vi "PopulatePrinterInitConfigDict.vi"(8 "error in (no error)":errorcluster, 11 "TopLevel in":refnum<class "TopLevel.lvclass">) -> (0 "error out":errorcluster, 3 "TopLevel out":refnum<class "TopLevel.lvclass">)   [LabVIEW 2022 SP3, in "TopLevel.lvclass"]
uses:
  TopLevel.lvclass
  Typedefs/PrinterHeads--Enum.ctl
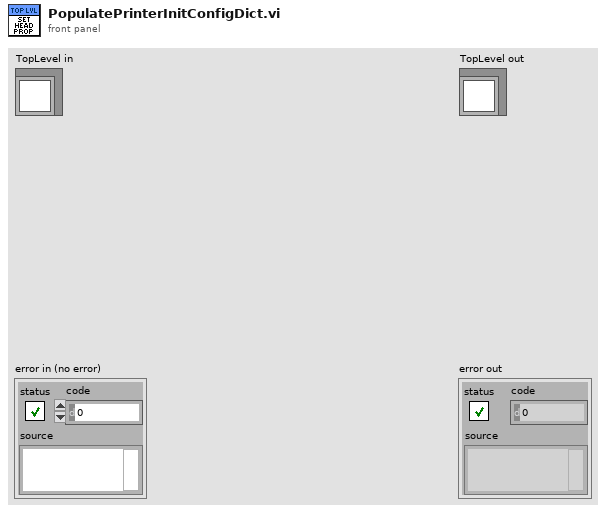
[diagram p1: front panel]
types:
  T1 = typedef "PrinterHeads--Enum.ctl" = enum16{"-1", "1", "2", "3", "4", "5", "6"}
  T2 = typedef "TD Dynamic CVT DVR--ref.ctl" = refnum<data-value>
  T3 = typedef "DLPConfig_Initialization.ctl" = cluster{"PrinterInitialization":cluster{"Printer":cluster{"#attributes":cluster{"Name":string}}, "VacPumpSet":cluster{"#attributes":cluster{"VacPumpEnable":bool, "VacPumpSpeed":dbl}}, "HIBEnable":cluster{"#attributes":cluster{"HIB1Enable":bool, "HIB2Enable":bool, "HIB3Enable":bool, "HIB4Enable":bool, "HIB5Enable":bool, "HIB6Enable":bool}}, "PrinterCompensation":T4}, "HeadSet":cluster{"HeadProperties":T5[]}, "InkSet":cluster{"Ink":T7[]}, "Troubleshooting":cluster{"PMBLogging":cluster{"#attributes":cluster{"PMBMonitorDuringPrint":bool, "PMBMonitorDuringIdle":bool, "LogSwatheInputData":bool, "LogSwatheOutputData":bool, "LogPrintheadColourPlanes":bool, "LogPMBCommunication":bool, "LogSimulatedOutput":bool, "LogAllPMBCommunicationData":bool, "LogPMBSpace":bool, "ExtendedPMBSpaceLogging":bool, "LogPMBWriteSpeed":bool, "LogUsbRetries":bool}}, "HIBLogging":cluster{"#attributes":cluster{"HIBMonitoringDuringPrint":bool, "HIBMonitoringLog":bool}}}}
  T4 = typedef "DLP2_PrinterCompensationProperties.ctl" = cluster{"#attributes":cluster{"AppName":string, "PrintWeightMultiplier":dbl, "Rotation":bool, "Driver":string, "Server":string, "Database":string, "User":string, "Password":string}}
  T5 = typedef "DLP2_PrinterHeadProperties.ctl" = cluster{"#attributes":T6}
  T6 = typedef "DLPConfig)Init_HeadPropertyAttr--Cluster.ctl" = cluster{"HeadNumber":u8, "Material":string, "HeadLocalX":dbl, "HeadLocalY":dbl, "HeadRotationAngle":dbl, "VH2L_Hi":dbl, "VH2R_Hi":dbl, "VH1LA_Hi":dbl, "VH1LB_Hi":dbl, "VH1RA_Hi":dbl, "VH1RB_Hi":dbl, "VH2L_Lo":dbl, "VH2R_Lo":dbl, "VH1LA_Lo":dbl, "VH1LB_Lo":dbl, "VH1RA_Lo":dbl, "VH1RB_Lo":dbl}
  T7 = typedef "DLP2_PrinterMaterialProperties.ctl" = cluster{"#attributes":cluster{"InkType":string, "PrePrintPurge":bool, "PurgeTime":dbl, "PurgeCount":i32, "Density":dbl, "NumberofDrops":i32, "PrintWeight":dbl, "PrintheadPrime":bool}, "Idle":cluster{"Name":string, "Heat":dbl, "Meniscus":dbl, "Recirculation":bool}[], "Process":cluster{"Name":string, "Heat":dbl, "Meniscus":dbl, "Recirculation":bool, "ColorPlane":string}[]}
  T8 = cluster{"HIB1Enable":bool, "HIB2Enable":bool, "HIB3Enable":bool, "HIB4Enable":bool, "HIB5Enable":bool, "HIB6Enable":bool}
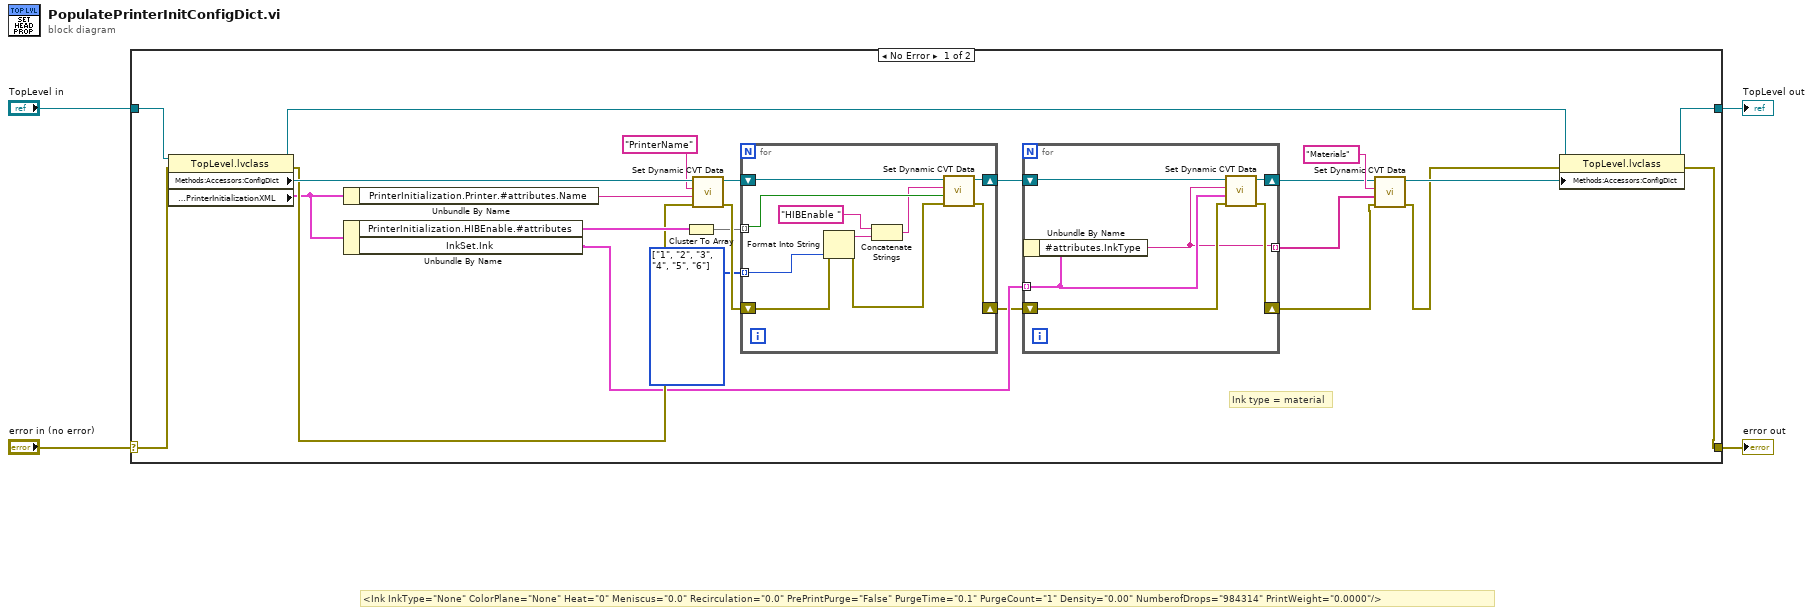
[diagram p0: block diagram]
diagram:
  # "<Ink InkType=\"None\" ColorPlane=\"None\" Heat=\"0\" Meniscus=\"0.0\" Recirculation=\"0.0\" PrePrintPurge=\"False\" PurgeTime=\"0.1\" PurgeCount=\"1\" Density=\"0.00\" NumberofDrops=\"984314\" PrintWeight=\"0.0000\"/>"
  n1 = case shown="No Error" "error in (no error)" {
    selector: "error in (no error)" -> [w23 w46]
    tunnel: [w22 w46] -> w3
    tunnel: [w27 w45] -> w1
    tunnel: "TopLevel in" -> [w24 w45]
    frame No Error {
      w14 = T1[] [enum."1", enum."2", enum."3", enum."4", enum."5", enum."6"] items=["-1", "1", "2", "3", "4", "5", "6"] ("Array")
      # "Ink type = material"
      n2 = property class="TopLevel.lvclass"(reference=w24, error in=w23) -> (reference out=w25:refnum<class "TopLevel.lvclass">, error out=w19:errorcluster, "Methods:Accessors:ConfigDict"=w28:T2, "Methods:Accessors:PrinterInitializationXML"=w16:T3)
      n3 = Unbundle By Name(w16) -> ("PrinterInitialization.Printer.#attributes.Name"=w26:string)
      n4 = Unbundle By Name(w16) -> ("PrinterInitialization.HIBEnable.#attributes"=w21:T8, "InkSet.Ink"=w12:T7[])
      n5 = Cluster To Array(cluster=w21) -> (array=w15:bool[])
      n6 = call <vilib>:"Set Dynamic CVT Data.vi"("error in (no error)"=w19, "value"=w26, "DataName"="PrinterName" ("string"), "dCVT DVR"=w28) -> ("error out"=w17:errorcluster, "dCVT DVR out"=w18:T2)  [unwired: 5 in, 1 out]
      n7 = for {
        tunnel: w15 -> [w41] mode=indexing
        shift-right: [w43] -> w13
        shift-left: w18 -> [w44]
        shift-right: [w42] -> w11
        shift-left: w17 -> [w36]
        tunnel: w14 -> [w35] mode=indexing
        n8 = Format Into String(error in=w36, w35) -> (resulting string=w39:string, error out=w37:errorcluster)  [unwired: 2 in]
        n9 = Concatenate Strings("HIBEnable " ("string"), w39) -> (w38:string)
        n10 = call <vilib>:"Set Dynamic CVT Data.vi"("error in (no error)"=w37, "value"=w41, "DataName"=w38, "dCVT DVR"=w44) -> ("error out"=w42:errorcluster, "dCVT DVR out"=w43:T2)  [unwired: 5 in, 1 out]
      }
      n11 = for {
        shift-right: [w33] -> w9
        shift-left: w13 -> [w34]
        shift-right: [w32] -> w7
        shift-left: w11 -> [w30]
        tunnel: w12 -> [w31] mode=indexing
        tunnel: [w29] -> w5 mode=indexing
        n12 = Unbundle By Name(w31) -> ("#attributes.InkType"=w29:string)
        n13 = call <vilib>:"Set Dynamic CVT Data.vi"("error in (no error)"=w30, "value"=w31, "DataName"=w29, "dCVT DVR"=w34) -> ("error out"=w32:errorcluster, "dCVT DVR out"=w33:T2)  [unwired: 5 in, 1 out]
      }
      n14 = call <vilib>:"Set Dynamic CVT Data.vi"("error in (no error)"=w7, "value"=w5, "DataName"="Materials" ("string"), "dCVT DVR"=w9) -> ("error out"=w6:errorcluster, "dCVT DVR out"=w8:T2)  [unwired: 5 in, 1 out]
      n15 = property class="TopLevel.lvclass"(reference=w25, error in=w6, "Methods:Accessors:ConfigDict"=w8) -> (reference out=w27:refnum<class "TopLevel.lvclass">, error out=w22:errorcluster)
    }
    frame Error {
    }
  }
  "error out" <- w3
  "TopLevel out" <- w1
